vi "Get Built Application Version from System.vi"(4 "Application Path (this application if blank)":path) -> (0 "LegalCopyright":string, 1 "Application Version (from System)":string)   [LabVIEW 2011]
doc: "This VI will return the system file version of a given application. If no application path is provided, the VI will get the Top Level VI path (which will be an .exe if built) and retrieve the system file version of that application instead."
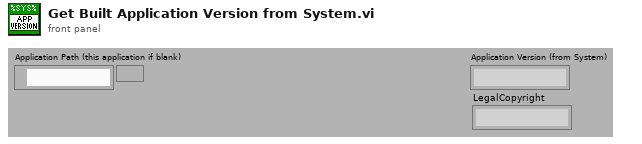
[diagram p1: front panel]
types:
  T1 = enum32{"invalid app kind", "Development System", "Run Time System", "Student Edition", "Embedded LabVIEW", "Evaluation", "Custom"}
  T2 = typedef "FileVersionInformation.ctl" = cluster{"FileVersion":string, "ProductName":string, "InternalName":string, "CompanyName":string, "LegalCopyright":string, "FileDescription":string}
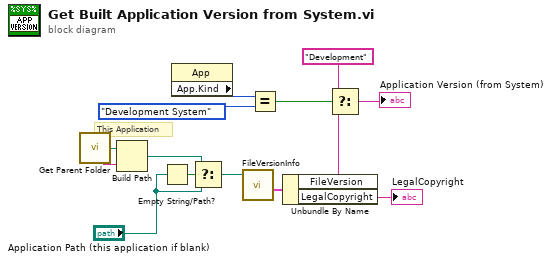
[diagram p0: block diagram]
diagram:
  # "This Application"
  n1 = call "Get Parent Folder.vi"() -> ("Top Level Filename"=w10:string, "path"=w11:path)  [unwired: 4 out]
  n2 = Build Path(base path=w11, name or relative path=w10) -> (appended path=w4:path)
  n3 = Empty String/Path?(string/path="Application Path (this application if blank)") -> (empty?=w5:bool)
  n4 = property class="App"() -> ("App.Kind"=w9:T1)  [unwired: 2 in, 2 out]
  n5 = Select(t=w4, s=w5, f="Application Path (this application if blank)") -> (s? t:f=w3:path)
  n6 = call <vilib>:"FileVersionInfo.vi"("Application Path in"=w3) -> ("FileVersionInfo Out"=w13:T2)  [unwired: 1 in, 9 out]
  n7 = Equal?(x=w9, y=T1."Development System" ("Application:Kind")) -> (x = y?=w7:bool)
  n8 = Unbundle By Name(w13) -> ("FileVersion"=w12:string, "LegalCopyright"=→"LegalCopyright":string)
  n9 = Select(t="Development", s=w7, f=w12) -> (s? t:f=→"Application Version (from System)":string)
